vi "Load Component User Interfaces.vi"(8 "error in (no error)":errorcluster, 10 "component names":string[](array[string]), 11 "Component Loader in":refnum<class "Component Loader.lvclass">) -> (0 "error out":errorcluster, 2 "Component UIs":refnum<class "Component User Interfaces.lvclass">[](array[class]), 3 "Component Loader out":refnum<class "Component Loader.lvclass">)   [LabVIEW 2017, in "DSF Core.lvlib" / "Component Loader.lvclass"]
uses:
  Component Loader.lvclass
  Component User Interface/Component User Interfaces.lvclass
  Component/Component.lvclass/Component.ctl
  Component Loader.lvclass/Component Loader.ctl
  Load Packed Library.vi
  Component/Create.vi
  Framework/Internal Components.vi
  Component/Get Name.vi
  Find Packed Library.vi
  Load Classes.vi
  Find Packed Library Classes.vi
  Component Configuration/Find.vi
  Component User Interface/Find.vi
  Find Packed Libraries.vi
  Errors.vi
  Component Not Found.vi
  Load Class.vi
  <vilib>/Utility/error.llb/Clear Errors.vi
  New Component Loader Error.vi
  Class Not Found.vi
  Component Loader Error Info.vi
  VIs/Constants/Constants.vi
  VIs/Constants/Engine Library Name.vi
  Base Error Offset.vi
  VIs/Constants/Base Error Code.vi
  <vilib>/Utility/LVClass/Get LV Class Default Value.vi
  <vilib>/NI/Memory Manager/VIs/Write String to Source.vi
  <vilib>/NI/Memory Manager/VIs/Set Error Source.vi
  <vilib>/NI/Memory Manager/VIs/Set Error Code.vi
  <vilib>/NI/Memory Manager/VIs/Set Error Status.vi
  <vilib>/NI/Memory Manager/VIs/New Error Cluster.vi
  <vilib>/NI/Memory Manager/VIs/New Error Cluster (512B).vi
  <vilib>/Utility/libraryn.llb/Check if File or Folder Exists.vi
  <vilib>/Utility/LVLibp/Get Exported File List.vi
  <vilib>/Utility/libraryn.llb/Recursive File List.vi
  Component Configuration/Component Configurations.lvclass
  Component/Component.lvclass
  Components/Buffer Converters/DSF Type Converter/DSF Buffer Converter.lvclass
  Components/Transceivers/UDP/UDP Transceiver.lvclass
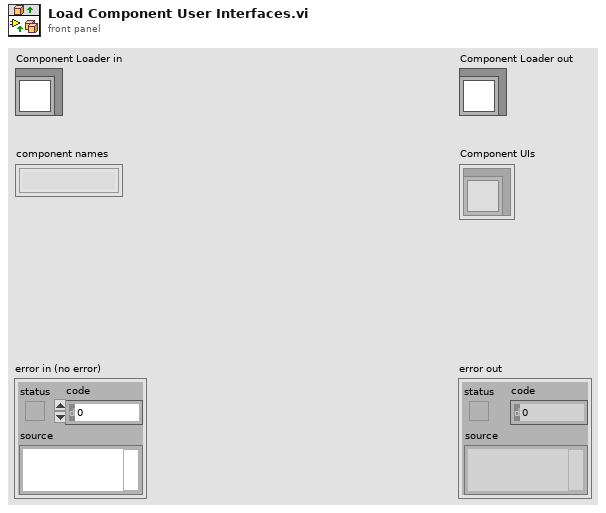
[diagram p1: front panel]
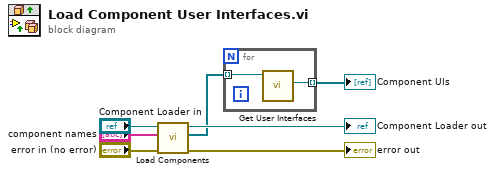
[diagram p0: block diagram]
diagram:
  n1 = call "Load Components.vi"("error in (no error)"="error in (no error)", "component names"="component names", "Component Loader in"="Component Loader in") -> ("error out"=→"error out":errorcluster, "Components"=w1:refnum<class "Component.lvclass">[], "Component Loader out"=→"Component Loader out":refnum<class "Component Loader.lvclass">)  [unwired: 6 in]
  n2 = for {
    tunnel: w1 -> [w9] mode=indexing
    tunnel: [w8] -> w2 mode=indexing
    n3 = call "Get User Interfaces.vi"("Component in"=w9) -> ("User Interfaces"=w8:refnum<class "Component User Interfaces.lvclass">)  [unwired: 9 in, 1 out]
  }
  "Component UIs" <- w2
